vi "transition.vi"(8 "error in (no error)":errorcluster, 10 "ContextData In":refnum<class "ContextData.lvclass">, 11 "Run in":refnum<class "Check Move.lvclass">) -> (0 "error out":errorcluster, 2 "ContextData Out":refnum<class "ContextData.lvclass">, 3 "Next Step":refnum<class "State.lvclass">)   [LabVIEW 2019, in "Check Move.lvclass"]
uses:
  Check Move.lvclass
  State/State.lvclass
  ContextData/ContextData.lvclass
  Wait Event/Wait Event.lvclass
  C:/Users/fflores/Documents/GitHub Projects/Simon/Simon Game/OOP States/State/State.lvclass
  Win/Win.lvclass
  Lost/Lost.lvclass
  Check Move.lvclass/Check Move.ctl
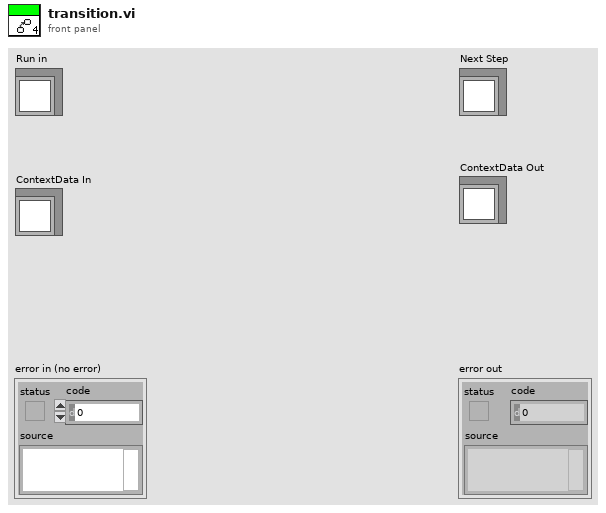
[diagram p1: front panel]
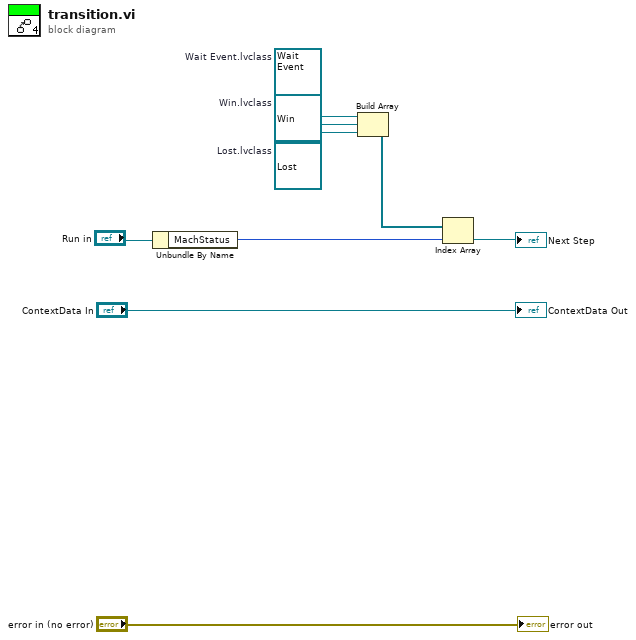
[diagram p0: block diagram]
diagram:
  w6 = refnum<class "Lost.lvclass"> refnum  # Lost.lvclass
  w7 = refnum<class "Win.lvclass"> refnum  # Win.lvclass
  w8 = refnum<class "Wait Event.lvclass"> refnum  # Wait Event.lvclass
  n1 = Unbundle By Name("Run in") -> ("MachStatus"=w1:i16)
  n2 = Build Array(w8, w7, w6) -> (w5:refnum<class "State.lvclass">[])
  n3 = Index Array(array=w5, index=w1) -> (element=→"Next Step":refnum<class "State.lvclass">)
  "error out" <- "error in (no error)"
  "ContextData Out" <- "ContextData In"
